vi "Calculate Scaling Factors.vi"(8 "error in (no error)":errorcluster, 11 "Pane Relief Main UI in":refnum<class "Pane Relief Main UI.lvclass">) -> (0 "error out":errorcluster, 3 "Pane Relief Main UI out":refnum<class "Pane Relief Main UI.lvclass">)   [LabVIEW 2015, in "Pane Relief Main UI.lvlib" / "Pane Relief Main UI.lvclass"]
uses:
  Pane Relief Main UI.lvclass
  Pane Relief Main UI.lvclass/Pane Relief Main UI.ctl
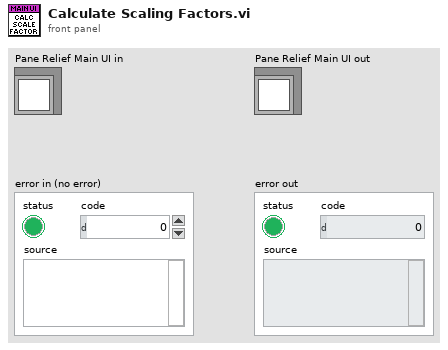
[diagram p1: front panel]
types:
  T1 = typedef "LVRectTypeDef.ctl" = cluster{"Left":i16, "Top":i16, "Right":i16, "Bottom":i16}
  T2 = typedef "LVBoundsTypeDef.ctl" = cluster{"Width":u32, "Height":u32}
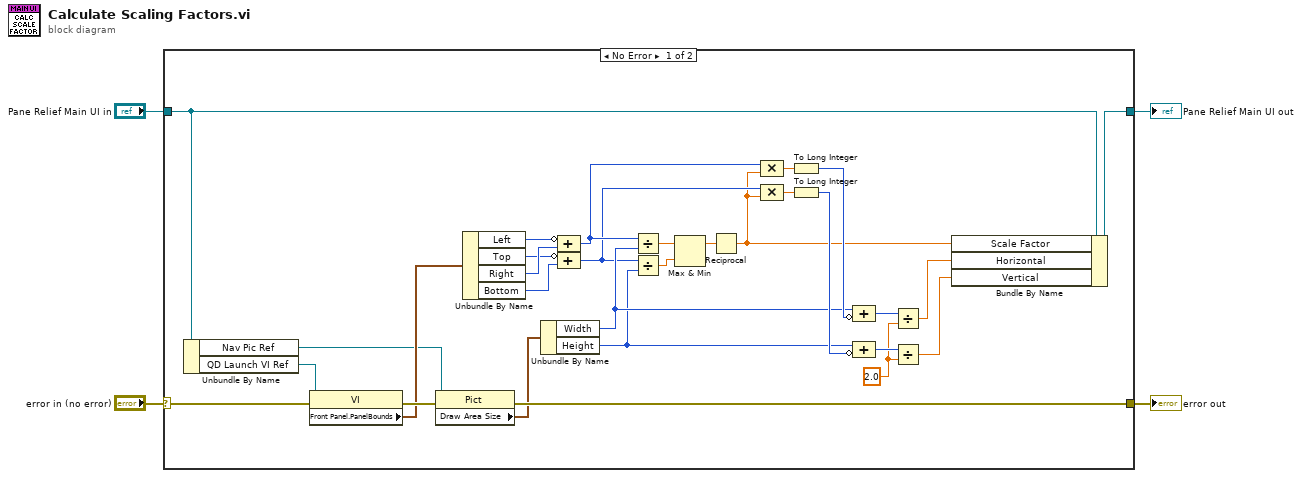
[diagram p0: block diagram]
diagram:
  n1 = case shown="No Error" "error in (no error)" {
    selector: "error in (no error)" -> [w13 w35]
    tunnel: [w12 w35] -> w3
    tunnel: "Pane Relief Main UI in" -> [w8 w36]
    tunnel: [w7 w36] -> w1
    frame No Error {
      w28 = 2.0 ("y")
      n2 = Unbundle By Name(w8) -> ("Nav Pic Ref"=w9:refnum<vi>, "QD Launch VI Ref"=w10:refnum<vi>)
      n3 = property class="VI"(reference=w10, error in=w13) -> (error out=w25:errorcluster, "Front Panel.PanelBounds"=w24:T1)  [unwired: 1 out]
      n4 = property on="Property Node" class="Pict"(reference=w9, error in=w25) -> (error out=w12:errorcluster, "Draw Area Size"=w5:T2)  [unwired: 1 out]
      n5 = Unbundle By Name(w24) -> ("Left"=w23:i16, "Top"=w21:i16, "Right"=w22:i16, "Bottom"=w20:i16)
      n6 = Unbundle By Name(w5) -> ("Width"=w19:u32, "Height"=w18:u32)
      n7 = Compound Arithmetic op=ADD(invert w23, w22) -> (w17:i16)
      n8 = Compound Arithmetic op=ADD(invert w21, w20) -> (w11:i16)
      n9 = Divide(x=w17, y=w19) -> (x/y=w16:dbl)
      n10 = Divide(x=w11, y=w18) -> (x/y=w15:dbl)
      n11 = Max & Min(x=w16, y=w15) -> (max(x,y)=w14:dbl)  [unwired: 1 out]
      n12 = Reciprocal(x=w14) -> (1/x=w6:dbl)
      n13 = Compound Arithmetic op=MULTIPLY(w17, w6) -> (w33:dbl)
      n14 = Compound Arithmetic op=MULTIPLY(w11, w6) -> (w34:dbl)
      n15 = To Long Integer(number=w33) -> (32bit integer=w32:i32)
      n16 = To Long Integer(number=w34) -> (32bit integer=w31:i32)
      n17 = Compound Arithmetic op=ADD(w19, invert w32) -> (w30:u32)
      n18 = Compound Arithmetic op=ADD(w18, invert w31) -> (w29:u32)
      n19 = Divide(x=w30, y=w28) -> (x/y=w27:dbl)
      n20 = Divide(x=w29, y=w28) -> (x/y=w26:dbl)
      n21 = Bundle By Name(cluster=w8, "Scale Factor"=w6, "Horizontal"=w27, "Vertical"=w26) -> (w7:refnum<class "Pane Relief Main UI.lvclass">)
    }
    frame Error {
    }
  }
  "error out" <- w3
  "Pane Relief Main UI out" <- w1
